vi "Get Terminal Owning Diagrams.vi"(8 "error in (no error)":errorcluster, 11 "Terminal in":refnum<vi>) -> (0 "error out":errorcluster, 1 "FlatSeqOutTun Refnum":refnum<vi>, 2 "FlatSeqInTun Refnum":refnum<vi>, 3 "Tunnel Ref":refnum<vi>, 4 "Terminal is on Tunnel":bool, 5 "Tunnel Type":enum16{"Tunnel", "FlatSeqInner", "FlatSeqOuter"}(ring), 7 "Owning Structure":refnum<vi>)   [LabVIEW 2023]
doc: "Returns one of three types of tunnel reference: normal structure tunnels; Inner and Outer tunnels of a flat sequence structure."
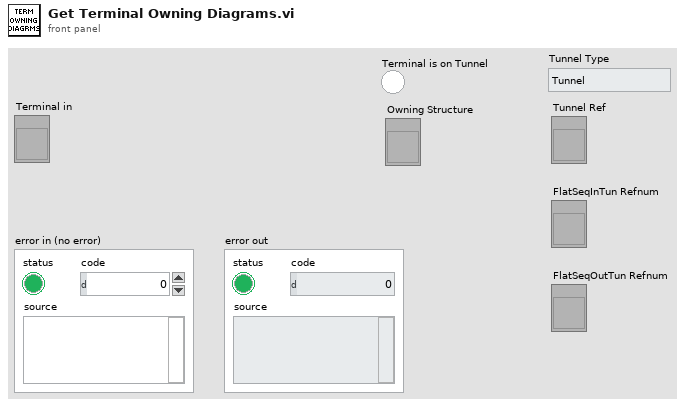
[diagram p1: front panel]
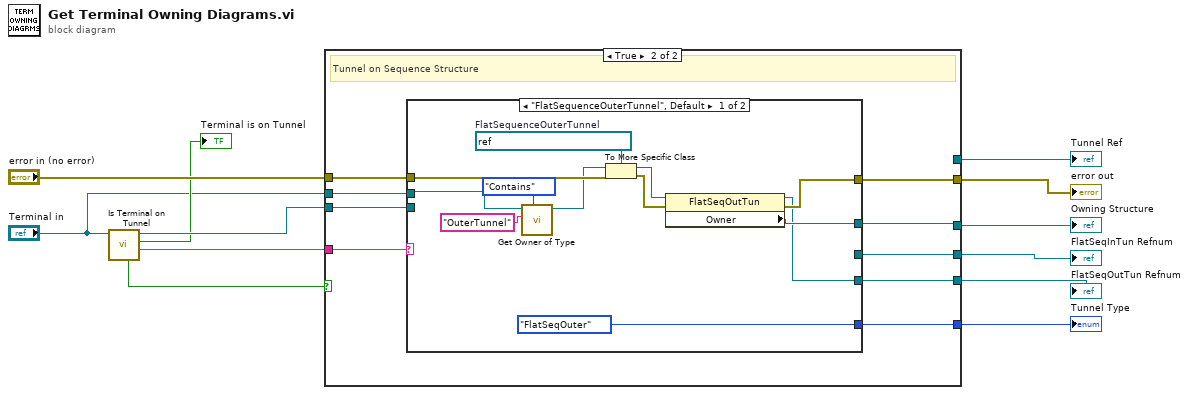
[diagram p0: block diagram]
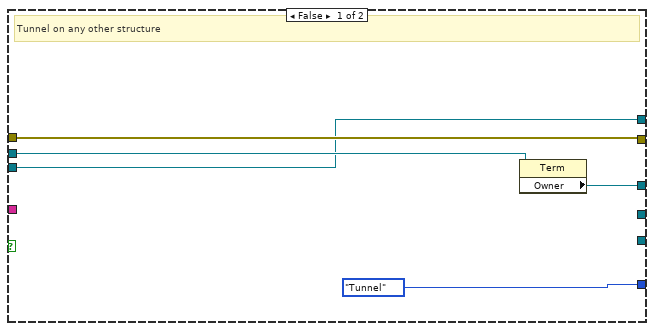
[diagram p2: hidden frame]
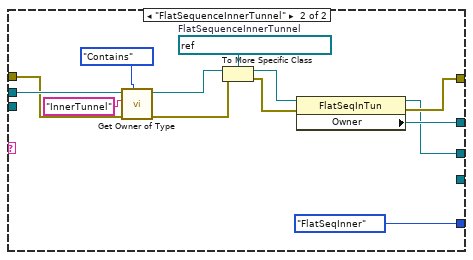
[diagram p3: hidden frame]
diagram:
  n1 = call "Is Terminal on Tunnel.vi"("Terminal in"="Terminal in") -> ("ClassName of tunnel ref"=w9:string, "Terminal is on Tunnel"=→"Terminal is on Tunnel":bool, "Tunnel Ref"=w10:refnum<vi>, "Tunnel on Flat Sequence?"=w8:bool)  [unwired: 4 in, 3 out]
  n2 = case shown="True" w8 {
    tunnel: [w15 w23] -> w12
    tunnel: "error in (no error)" -> [w15 w24]
    tunnel: w10 -> [w13 w25]
    tunnel: w9 -> [_ w26]
    tunnel: [_ w22] -> w7
    tunnel: [_ w21] -> w6
    tunnel: [enum16{"Tunnel", "FlatSeqInner", "FlatSeqOuter"}."Tunnel" ("Tunnel Type") w20] -> w5
    tunnel: [w16 w19] -> w4
    tunnel: "Terminal in" -> [w14 w18]
    tunnel: [w13 _] -> w1
    frame False {
      # "Tunnel on any other structure"
      n3 = property class="Term"(reference=w14) -> ("Owner"=w16:refnum<vi>)  [unwired: 1 in, 2 out]
    }
    frame True {
      # "Tunnel on Sequence Structure"
      n4 = case shown="\"FlatSequenceOuterTunnel\", Default" w26 {
        tunnel: w25 -> [_ _]
        tunnel: w24 -> [w37 w39]
        tunnel: [w33 w48] -> w23
        tunnel: [_ w46] -> w22
        tunnel: [w32 _] -> w21
        tunnel: [enum16{"Tunnel", "FlatSeqInner", "FlatSeqOuter"}."FlatSeqOuter" ("Tunnel Type") enum16{"Tunnel", "FlatSeqInner", "FlatSeqOuter"}."FlatSeqInner" ("Tunnel Type")] -> w20
        tunnel: [w35 w47] -> w19
        tunnel: w18 -> [w29 w42]
        frame "FlatSequenceOuterTunnel", Default {
          w38 = refnum<vi> refnum  # FlatSequenceOuterTunnel
          n5 = call "Get Owner of Type.vi"("Match Type"=enum16{"Exact Match", "Contains"}."Contains", "Owner Class Name desired"="OuterTunnel", "reference"=w29) -> ("Owner of Type"=w28:refnum<vi>)  [unwired: 4 in, 4 out]
          n6 = To More Specific Class(target class=w38, reference=w28, error in=w37) -> (specific class reference=w31:refnum<vi>, error out=w34:errorcluster)
          n7 = property class="FlatSeqOutTun"(reference=w31, error in=w34) -> (reference out=w32:refnum<vi>, error out=w33:errorcluster, "Owner"=w35:refnum<vi>)
        }
        frame "FlatSequenceInnerTunnel" {
          w51 = refnum<vi> refnum  # FlatSequenceInnerTunnel
          n8 = call "Get Owner of Type.vi"("Match Type"=enum16{"Exact Match", "Contains"}."Contains", "error in"=w39, "Owner Class Name desired"="InnerTunnel", "reference"=w42) -> ("error out"=w40:errorcluster, "Owner of Type"=w41:refnum<vi>)  [unwired: 3 in, 3 out]
          n9 = To More Specific Class(target class=w51, reference=w41, error in=w40) -> (specific class reference=w45:refnum<vi>, error out=w49:errorcluster)
          n10 = property class="FlatSeqInTun"(reference=w45, error in=w49) -> (reference out=w46:refnum<vi>, error out=w48:errorcluster, "Owner"=w47:refnum<vi>)
        }
      }
    }
  }
  "Tunnel Ref" <- w1
  "error out" <- w12
  "FlatSeqInTun Refnum" <- w7
  "FlatSeqOutTun Refnum" <- w6
  "Tunnel Type" <- w5
  "Owning Structure" <- w4
